vi "SubVI_Status.vi"(8 "error in (no error)":errorcluster caption="err in", 11 "info_str":string) -> (0 "error out":errorcluster caption="err out")   [LabVIEW 2016]
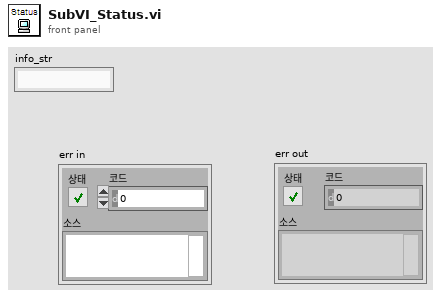
[diagram p1: front panel]
types:
  T1 = typedef "ui ctrl ref2.ctl" = cluster{"Trigger cm":refnum<vi>, "Speed In/s":refnum<vi>, "Start / Stop":refnum<vi>, "Test Information":refnum<vi>, "STATUS":refnum<vi>, "Result Table":refnum<vi>, "Acc. & Strian Result":refnum<vi>, "Curr Resistor (Ω)":refnum<vi>, "Scroll":refnum<vi>, "All Data Graph":refnum<vi>, "Acc. Graph":refnum<vi>}
  T2 = cluster{"status":string, "all_fail":bool, "emg":bool, "cycle":u16, "file name":string, "Total Cycle":u32}
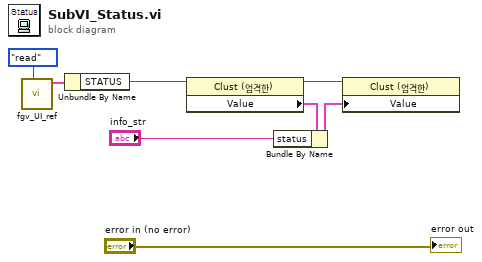
[diagram p0: block diagram]
diagram:
  n1 = call "fgv_UI_ref.vi"("cmd"=enum16{"write", "read"}."read") -> ("ui ref out"=w3:T1)  [unwired: 10 in]
  n2 = Unbundle By Name(w3) -> ("STATUS"=w7:refnum<vi>)
  n3 = property class="Clust (엄격한)"(reference=w7) -> (reference out=w6:refnum<vi>, "Value"=w4:T2)  [unwired: 1 in, 1 out]
  n4 = Bundle By Name(cluster=w4, "status"="info_str") -> (w5:T2)
  n5 = property class="Clust (엄격한)"(reference=w6, "Value"=w5) -> ()  [unwired: 1 in, 2 out]
  "error out" <- "error in (no error)"
